vi "steps.util.findStepByLabel.vi"(6 "isRequired?(T)":bool=TRUE, 8 "error":errorcluster, 10 "stepLabel":string, 11 "steps in":variant[](array[variant])) -> (0 "error":errorcluster, 3 "index":i32)   [LabVIEW 2024]
uses:
  controls/typeStepVarients.ctl
  Polymorphics/variantCtrlString.vi
  proc.util.validateParamExist.vi
  <vilib>/Utility/error.llb/Clear Errors.vi
  util.error.create.vi
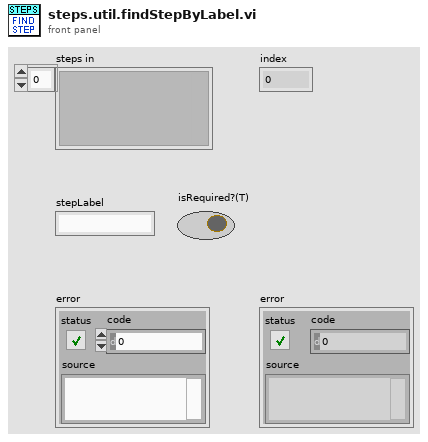
[diagram p1: front panel]
types:
  T1 = typedef "typeStepVarients.ctl" = enum16{"stepNameID", "stepFunction", "stepReport", "stepSetpoint", "stepPointer", "stepProcPointer", "stepIoPointer", "stepIoValue", "stepFilePointer", "stepMessage", "stepTimeString", "stepNumReg", "stepStrReg", "stepSeconds", "stepUnitDoseParams", "stepUnitIndex"}
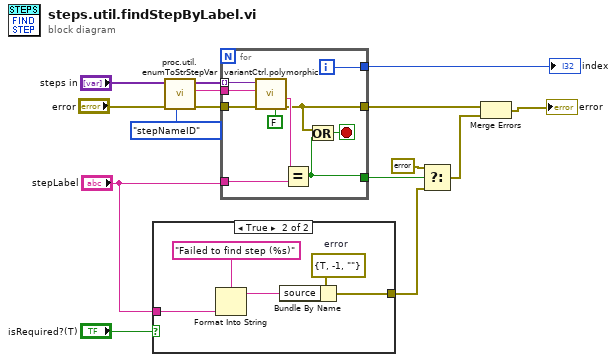
[diagram p0: block diagram]
diagram:
  n1 = case shown="True" "isRequired?(T)" {
    tunnel: "stepLabel" -> [_ w17]
    tunnel: [_ w14] -> w1
    frame False {
    }
    frame True {
      w16 = errorcluster {"status"=TRUE, "code"=-1, "source"=""}  # error
      n2 = Format Into String(format string="Failed to find step (%s)" ("source"), w17) -> (resulting string=w15:string)  [unwired: 2 in, 1 out]
      n3 = Bundle By Name(cluster=w16, "source"=w15) -> (w14:errorcluster)
    }
  }
  n4 = call "proc.util.enumToStrStepVar.vi"("Step var"=typeStepVarients."stepNameID" ("proc var")) -> ("String"=w11:string)  [unwired: 10 in]
  n5 = for {
    tunnel: "steps in" -> [w19] mode=indexing
    tunnel: "stepLabel" -> [w27]
    tunnel: [w26] -> w8
    tunnel: [w25] -> w10
    tunnel: "error" -> [w24]
    tunnel: [w22] -> w5
    tunnel: w11 -> [w21]
    i -> [w26]
    stop <- w23 stop-if-true
    n6 = call-poly "variantCtrl.polymorphic.vi"("isRequired (T)"=FALSE, "error in"=w24, "name in"=w21, "Step in"=w19) -> ("error out"=w22:errorcluster, "String Value"=w28:string)  [unwired: 4 in, 2 out]
    n7 = Equal?(x=w28, y=w27) -> (x = y?=w25:bool)
    n8 = Or(x=w22, y=w25) -> (x .or. y?=w23:bool)
  }
  "index" <- w8
  n9 = Select(t=errorcluster {"status"=FALSE, "code"=0, "source"=""}, s=w10, f=w1) -> (s? t:f=w13:errorcluster)
  n10 = Merge Errors(w5, w13) -> (→"error":errorcluster)
